vi "Deneme Counter.vi"() -> ()   [LabVIEW 2019]
panel:
  in  "Enum":T1(ring)
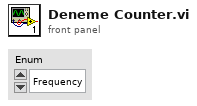
[diagram p1: front panel]
types:
  T1 = enum16{"Frequency", "Period", "Semi-Period", "Pulse Width", "Count", "Wait for Event"}
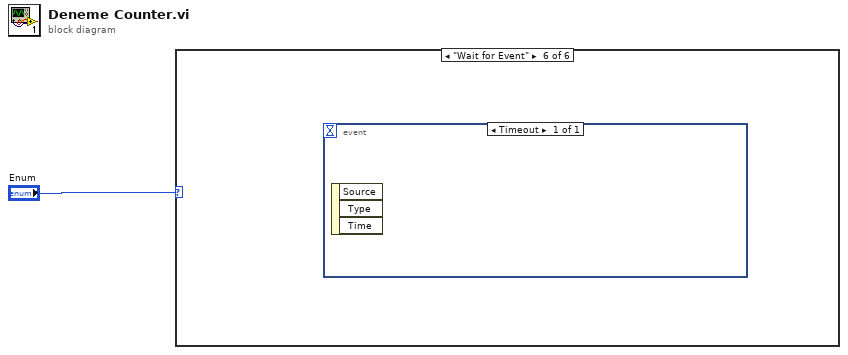
[diagram p0: block diagram]
diagram:
  n1 = case shown="\"Wait for Event\"" "Enum" {
    frame "Frequency", Default {
    }
    frame "Period" {
    }
    frame "Semi-Period" {
    }
    frame "Pulse Width" {
    }
    frame "Count" {
    }
    frame "Wait for Event" {
      n2 = event shown="[0] Timeout" {
        selector: _ -> [_]
        dyn-events: _ -> [_]
        timeout: _ -> [_]
        event Timeout {
          n3 = event-data() -> ()  [unwired: 1 in, 3 out]
        }
      }
    }
  }
